vi "State exit CONSTANT.vi"() -> (0 "Exit state":string)   [LabVIEW 2013, in "State Machine Lib.lvlib"]
doc: "Used to build and parse state hierarchies."
uses:
  State Machine Lib.lvlib
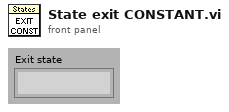
[diagram p1: front panel]
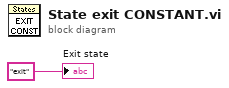
[diagram p0: block diagram]
diagram:
  "Exit state" <- "exit" ("regular expression")
